vi "test_Util_CalculateDistanceToTarget.vi"(8 "error in (no error)":errorcluster) -> (0 "error out":errorcluster, 3 "Test Passed":bool)   [LabVIEW 2019]
uses:
  <vilib>/Rock Robotics/WPI/ThirdParty/PhotonVisionLib/PhotonVisionLib.lvlib
  <vilib>/Rock Robotics/WPI/ThirdParty/JAS_Junk/TrajLib/Trajectory_Library.lvlib
panel:
  out "T1 Dist":dbl
  out "T0 Dist":dbl
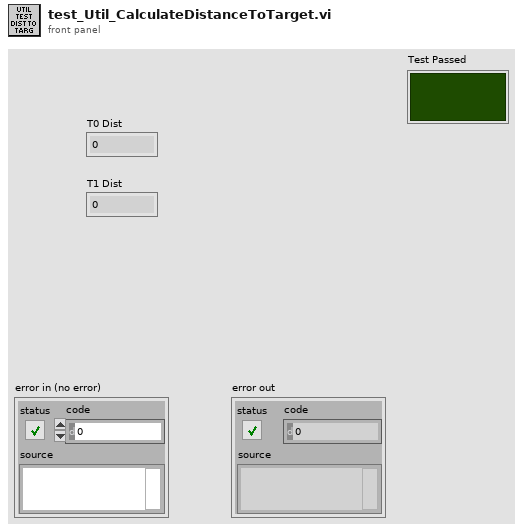
[diagram p1: front panel]
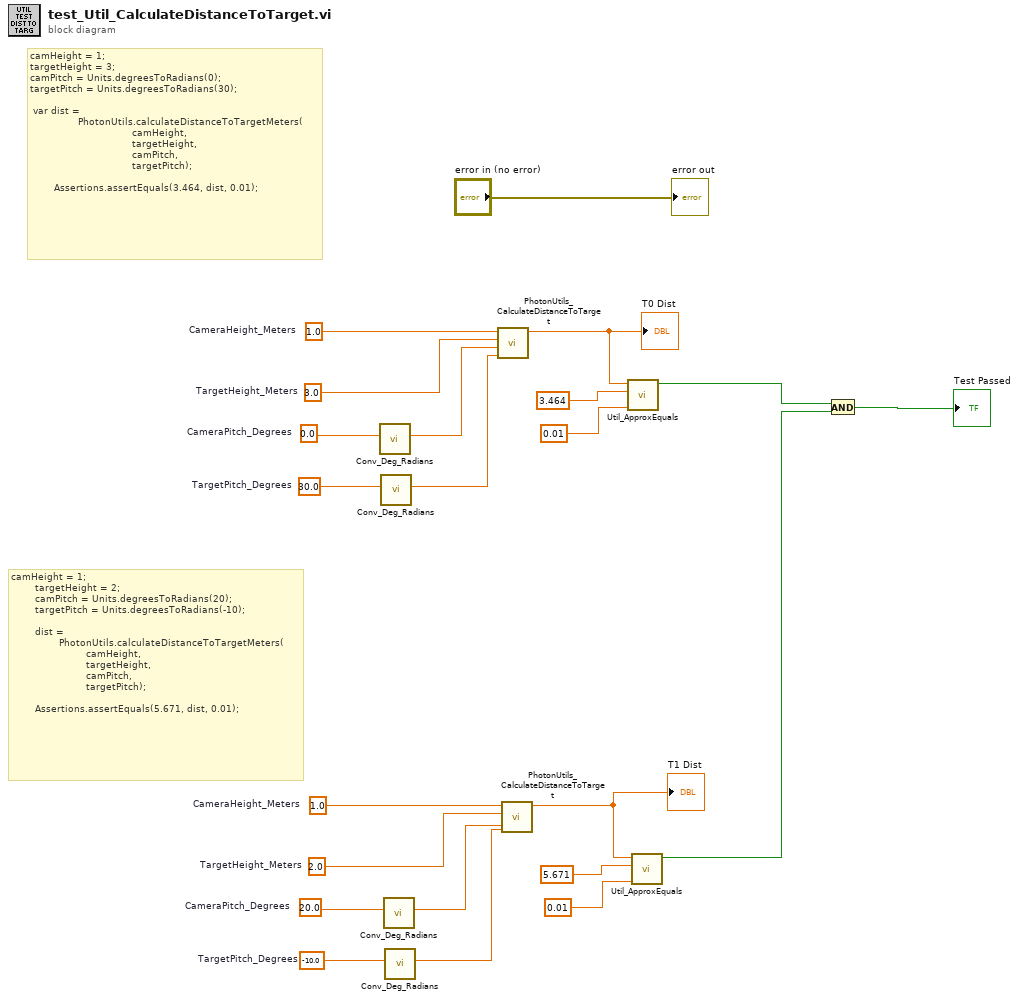
[diagram p0: block diagram]
diagram:
  w9 = 1.0  # CameraHeight_Meters
  w10 = 2.0  # TargetHeight_Meters
  w8 = 20.0  # CameraPitch_Degrees
  w7 = -10.0  # TargetPitch_Degrees
  w21 = 1.0  # CameraHeight_Meters
  w22 = 3.0  # TargetHeight_Meters
  w20 = 0.0  # CameraPitch_Degrees
  w19 = 30.0  # TargetPitch_Degrees
  # "camHeight = 1;\n        targetHeight = 2;\n        camPitch = Units.degreesToRadians(20);\n        targetPitch = Units.degreesToRadians(-10);\n\n        dist =\n                PhotonUtils.calculateDistanceToTargetMeters(\n                         camHeight, \n                         targetHeight, \n                         camPitch, \n                         targetPitch);\n\n        Assertions.assertEquals(5.671, dist, 0.01);"
  # "camHeight = 1;\ntargetHeight = 3;\ncamPitch = Units.degreesToRadians(0);\ntargetPitch = Units.degreesToRadians(30);\n\n var dist =\n                PhotonUtils.calculateDistanceToTargetMeters(\n                                  camHeight, \n                                  targetHeight, \n                                  camPitch, \n                                  targetPitch);\n\n        Assertions.assertEquals(3.464, dist, 0.01);"
  n1 = call <vilib>:"Conv_Deg_Radians.vi"("Degress"=w20) -> ("Radians"=w18:dbl)  [unwired: 10 in]
  n2 = call <vilib>:"Conv_Deg_Radians.vi"("Degress"=w19) -> ("Radians"=w17:dbl)  [unwired: 10 in]
  n3 = call <vilib>:"Conv_Deg_Radians.vi"("Degress"=w8) -> ("Radians"=w6:dbl)  [unwired: 10 in]
  n4 = call <vilib>:"Conv_Deg_Radians.vi"("Degress"=w7) -> ("Radians"=w5:dbl)  [unwired: 10 in]
  n5 = call <vilib>:"PhotonUtils_CalculateDistanceToTarget.vi"("TargetPitch_Radians"=w17, "CameraPitch_Radians"=w18, "TargetHeight_Meters"=w22, "CameraHeight_Meters"=w21) -> ("DistanceToTarget_Meters"=w16:dbl)  [unwired: 7 in]
  "T0 Dist" <- w16
  n6 = call <vilib>:"PhotonUtils_CalculateDistanceToTarget.vi"("TargetPitch_Radians"=w5, "CameraPitch_Radians"=w6, "TargetHeight_Meters"=w10, "CameraHeight_Meters"=w9) -> ("DistanceToTarget_Meters"=w1:dbl)  [unwired: 7 in]
  "T1 Dist" <- w1
  n7 = call <vilib>:"Util_ApproxEquals.vi"("Tolerance"=0.01, "Value 2"=3.464, "Value 1"=w16) -> ("ApproxEquals"=w13:bool)  [unwired: 8 in]
  n8 = call <vilib>:"Util_ApproxEquals.vi"("Tolerance"=0.01, "Value 2"=5.671, "Value 1"=w1) -> ("ApproxEquals"=w2:bool)  [unwired: 8 in]
  n9 = And(x=w13, y=w2) -> (x .and. y?=→"Test Passed":bool)
  "error out" <- "error in (no error)"
